vi "Array Control to Key List.vi"(5 "section":string, 7 "Prefix":string, 8 "Error In":errorcluster, 11 "Ctl Refnum":refnum<vi>) -> (0 "Error Out":errorcluster, 3 "Ctl Refnum out":refnum<vi>)   [LabVIEW 2015]
uses:
  <vilib>/Utility/Data Type/NI_Data Type.lvlib
panel:
  in  "Numberof lements":i32
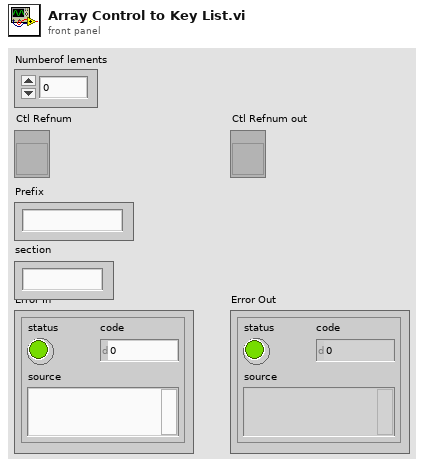
[diagram p1: front panel]
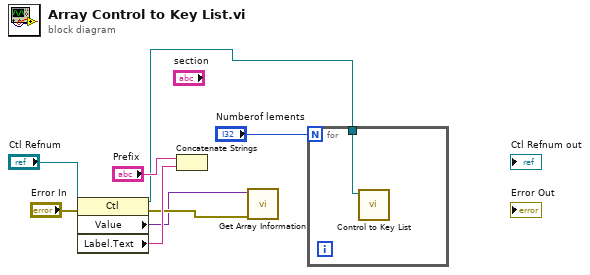
[diagram p0: block diagram]
diagram:
  n1 = property class="Ctl"(reference="Ctl Refnum", error in="Error In") -> (reference out=w2:refnum<vi>, error out=w5:errorcluster, "Value"=w3:variant, "Label.Text"=w6:string)
  n2 = Concatenate Strings("Prefix", w6) -> ()  [unwired: 1 out]
  n3 = call <vilib>:"Get Array Information.vi"("error in (no error)"=w5, "Variant"=w3) -> ()  [unwired: 6 in, 4 out]
  n4 = for {
    N: "Numberof lements" -> [_]
    tunnel: w2 -> [w9]
    n5 = call "Control to Key List.vi"("Ctl Refnum"=w9) -> ()  [unwired: 9 in, 2 out]
  }
